vi "Teleop.vi"(10 "Match Info":T1={"Autonomous Elapsed Seconds"=0.0, "TeleOp Elapsed Seconds"=0.0, "Disabled Elapsed Seconds"=0.0, "Visited Autonomous"=FALSE, "Visited TeleOp"=FALSE, "Visited Disabled"=FALSE, "Autonomous Settings"={"Autonomous Style"=enum."Independent", "VI Refnum"=refnum}}, 11 "Call Context":T2) -> ()   [LabVIEW 2016]
doc: "This VI is called for each TeleOp packet received from the DS where the robot is not disabled. It is often used to read from the joysticks and update I/O or to update setpoints for timed control loops. It should complete and return within 20 milliseconds or it may miss DS packets."
uses:
  <vilib>/Rock Robotics/WPI/DriverStation/WPI_DriverStationDerivedRobotMode.ctl
  <vilib>/Rock Robotics/WPI/DriverStation/WPI_DriverStationMatch Info.ctl
  <vilib>/Rock Robotics/WPI/Solenoid/WPI_SolenoidValue.ctl
  <vilib>/Rock Robotics/Network Tables/NT Read Boolean.vi
  <vilib>/Rock Robotics/Network Tables/NT Read Number.vi
  <vilib>/Rock Robotics/WPI/Utilities/WPI_GetSetVariantRefNum.vi
  <vilib>/Rock Robotics/WPI/Solenoid/WPI_SolenoidSetEnum.vi
panel:
  out "Teleop Time Elipsed":dbl
  in  "Quand arreter compresseur":dbl
  out "Droit":dbl
  out "Gauche":dbl
  out "Corde start time":dbl
  out "Sample Slider 0":dbl(slide) scale=0.0..5.0
  out "Sample Boolean 1":bool
  out "Sample Boolean 0":bool
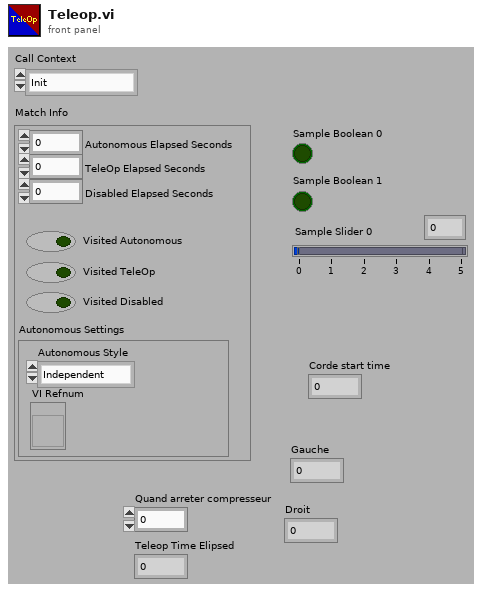
[diagram p1: front panel]
types:
  T1 = typedef "WPI_DriverStationMatch Info.ctl" = cluster{"Autonomous Elapsed Seconds":dbl, "TeleOp Elapsed Seconds":dbl, "Disabled Elapsed Seconds":dbl, "Visited Autonomous":bool, "Visited TeleOp":bool, "Visited Disabled":bool, "Autonomous Settings":cluster{"Autonomous Style":enum16{"Iterative", "Independent"}, "VI Refnum":refnum<vi>}}
  T2 = typedef "WPI_DriverStationDerivedRobotMode.ctl" = enum16{"Init", "Execute", "Stop"}
  T3 = typedef "WPI_SolenoidValue.ctl" = enum16{"Off", "On", "Forward", "Reverse"}
  T4 = typedef "WPI_JoystickDevRef.ctl" = cluster{"Device":T5}
  T5 = typedef "WPI_JoystickDeviceEnum.ctl" = enum16{"USB 0", "USB 1", "USB 2", "USB 3", "USB 4", "USB 5"}
  T6 = typedef "WPI_EncoderDevRef.ctl" = cluster{"DevStatus":errorcluster, "EncoderIndex":T7, "CounterIndex":T8, "DistancePerCount":dbl, "Decoding Type":T9}
  T7 = typedef "FPGA_EncoderIdx.ctl" = enum8{"Enc 0", "Enc 1", "Enc 2", "Enc 3", "Enc 4", "Enc 5", "Enc 6", "Enc 7", "Invalid"}
  T8 = typedef "FPGA_CounterCtrSystemIndex.ctl" = enum8{"Ctr 0", "Ctr 1", "Ctr 2", "Ctr 3", "Ctr 4", "Ctr 5", "Ctr 6", "Ctr 7", "Invalid"}
  T9 = typedef "WPI_EncoderType.ctl" = enum16{"1x", "2x", "4x"}
  T10 = cluster{"Buttons[0]":bool, "Buttons[1]":bool, "Buttons[2]":bool, "Buttons[3]":bool, "Buttons[4]":bool, "Buttons[5]":bool, "Buttons[6]":bool, "Buttons[7]":bool, "Buttons[8]":bool}
  T11 = cluster{"Axes[0]":dbl, "Axes[1]":dbl, "Axes[2]":dbl, "Axes[3]":dbl, "Axes[4]":dbl, "Axes[5]":dbl, "Axes[6]":dbl, "Axes[7]":dbl, "Axes[8]":dbl}
  T12 = typedef "WPI_RobotDriveDevRef.ctl" = cluster{"DevStatus":errorcluster, "Motors[]":T13[], "Square Inputs":bool, "Max Output":dbl}
  T13 = typedef "WPI_MotorControlDeviceRef.ctl" = cluster{"DeviceStatus":errorcluster, "Type":T14, "PWM":cluster{"PWM Channel":T15, "DeadBand":T16}, "CAN":cluster{"Device Number":u8, "SetOutput VI Ref":variant, "GetOutput VI Ref":variant, "Enable VI Ref":variant, "Disable VI Ref":variant, "Data":variant}, "Invert":bool}
  T14 = typedef "WPI_MotorControlType.ctl" = enum16{"PWM", "CAN"}
  T15 = typedef "FPGA_DIOPWMChannel.ctl" = enum8{"PWM 0", "PWM 1", "PWM 2", "PWM 3", "PWM 4", "PWM 5", "PWM 6", "PWM 7", "PWM 8", "PWM 9", "PWM MXP 0", "PWM MXP 1", "PWM MXP 2", "PWM MXP 3", "PWM MXP 4", "PWM MXP 5", "PWM MXP 6", "PWM MXP 7", "PWM MXP 8", "PWM MXP 9", "Invalid"}
  T16 = typedef "WPI_PWMDeadband.ctl" = cluster{"Name":string, "maxPositivePwm":i32, "minPositivePwm":i32, "centerPwm":i32, "maxNegativePwm":i32, "minNegativePwm":i32, "angularRange":u16}
  T17 = typedef "WPI_SolenoidDevRef.ctl" = cluster{"DevStatus":errorcluster, "Pneumatics Control Module":u8, "Forward Solenoid Channel":T18, "Reverse Solenoid Channel":T18}
  T18 = typedef "WPI_SolenoidChannel.ctl" = enum8{"Solenoid 0", "Solenoid 1", "Solenoid 2", "Solenoid 3", "Solenoid 4", "Solenoid 5", "Solenoid 6", "Solenoid 7", "Invalid"}
  T19 = typedef "WPI_CompressorDevRef.ctl" = cluster{"DevStatus":errorcluster, "Pneumatics Control Module":u8}
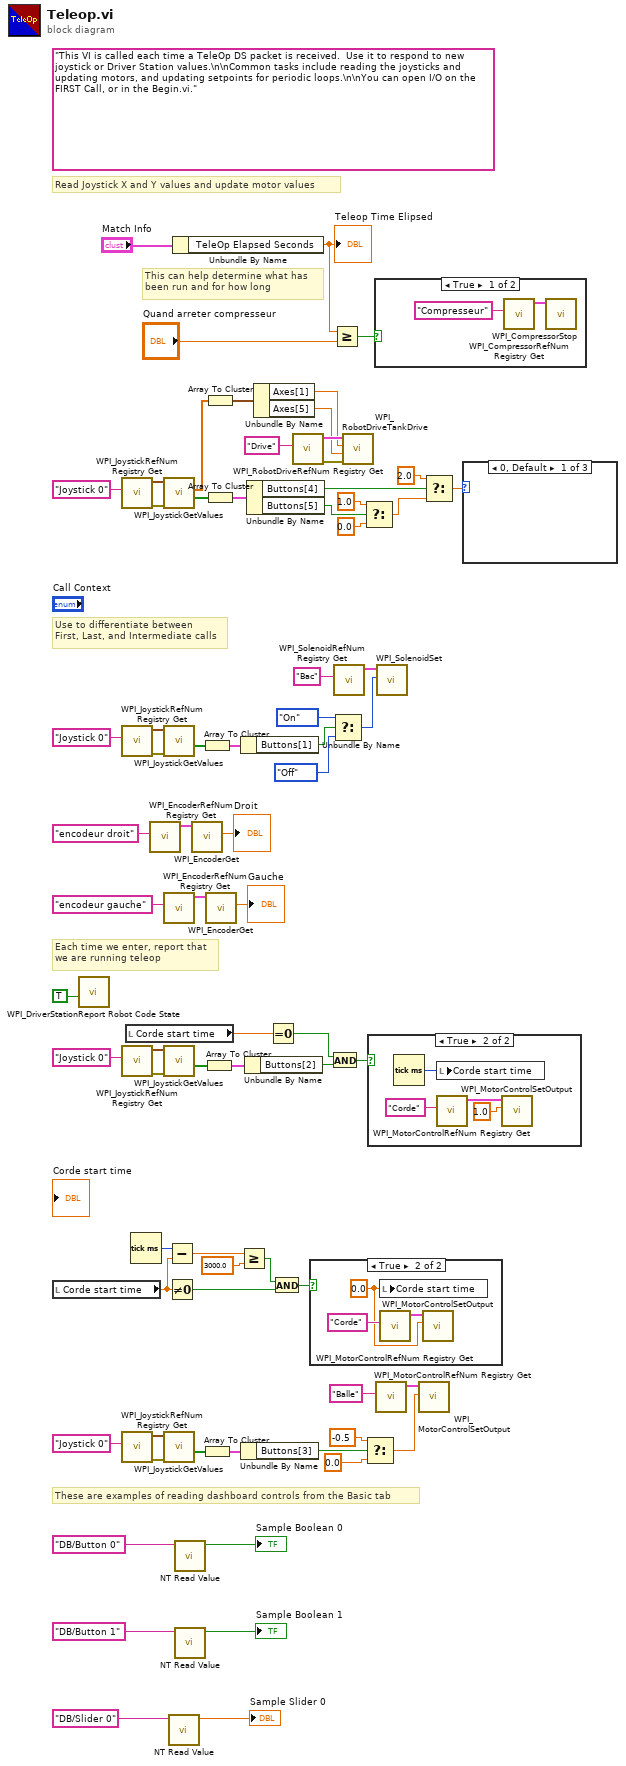
[diagram p0: block diagram]
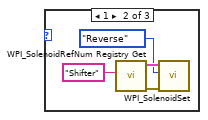
[diagram p5: hidden frame]
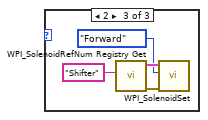
[diagram p6: hidden frame]
diagram:
  (unwired) "This VI is called each time a TeleOp DS packet is received.  Use it to respond to new joystick or Driver Station values.\n\nCommon tasks include reading the joysticks and updating motors, and updating setpoints for periodic loops.\n\nYou can open I/O on the FIRST Call, or in the Begin.vi."
  # "These are examples of reading dashboard controls from the Basic tab"
  # "Each time we enter, report that\nwe are running teleop"
  # "Use to differentiate between\nFirst, Last, and Intermediate calls"
  # "This can help determine what has\nbeen run and for how long"
  # "Read Joystick X and Y values and update motor values"
  n1 = local read "Corde start time"() -> (w10:dbl)
  n2 = call <vilib>:"WPI_DriverStationReport Robot Code State.vi"("TeleOp"=TRUE ("Autonomous")) -> ()  [unwired: 10 in, 1 out]
  n3 = call <vilib>:"WPI_JoystickRefNum Registry Get.vi"("refnum name"="Joystick 0") -> ("error out"=w63:errorcluster, "JoystickDevRef"=w62:T4)  [unwired: 9 in]
  n4 = call <vilib>:"WPI_JoystickRefNum Registry Get.vi"("refnum name"="Joystick 0") -> ("error out"=w47:errorcluster, "JoystickDevRef"=w48:T4)  [unwired: 1 in, 8 out]
  n5 = call <vilib>:"WPI_JoystickRefNum Registry Get.vi"("refnum name"="Joystick 0") -> ("error out"=w36:errorcluster, "JoystickDevRef"=w37:T4)  [unwired: 1 in, 8 out]
  n6 = call <vilib>:"WPI_JoystickRefNum Registry Get.vi"("refnum name"="Joystick 0") -> ("error out"=w31:errorcluster, "JoystickDevRef"=w32:T4)  [unwired: 1 in, 8 out]
  n7 = local read "Corde start time"() -> (w17:dbl)
  n8 = Tick Count (ms)() -> (millisecond timer value=w16:u32)
  n9 = call <vilib>:"WPI_EncoderRefNum Registry Get.vi"("refnum name"="encodeur droit") -> ("EncoderDevRef"=w8:T6)  [unwired: 9 in, 1 out]
  n10 = call <vilib>:"WPI_JoystickGetValues.vi"("error in (no error)"=w63, "JoystickDevRef"=w62) -> ("Buttons"=w58:bool[], "Axes"=w61:dbl[])  [unwired: 5 in, 3 out]
  n11 = call <vilib>:"WPI_JoystickGetValues.vi"("error in (no error)"=w47, "JoystickDevRef"=w48) -> ("Buttons"=w46:bool[])  [unwired: 5 in, 4 out]
  n12 = call <vilib>:"WPI_EncoderRefNum Registry Get.vi"("refnum name"="encodeur gauche") -> ("EncoderDevRef"=w9:T6)  [unwired: 9 in, 1 out]
  n13 = call <vilib>:"WPI_JoystickGetValues.vi"("error in (no error)"=w36, "JoystickDevRef"=w37) -> ("Buttons"=w35:bool[])  [unwired: 5 in, 4 out]
  n14 = call <vilib>:"WPI_JoystickGetValues.vi"("error in (no error)"=w31, "JoystickDevRef"=w32) -> ("Buttons"=w30:bool[])  [unwired: 5 in, 4 out]
  n15 = Subtract(x=w16, y=w10) -> (x-y=w15:dbl)
  n16 = Not Equal To 0?(x=w10) -> (x != 0?=w12:bool)
  n17 = call-poly <vilib>:"NT Read Value.vi"("Name"="DB/Slider 0" ("refnum name")) -> ("Numeric"=→"Sample Slider 0":dbl)  [unwired: 9 in, 1 out]
  n18 = Unbundle By Name("Match Info") -> ("TeleOp Elapsed Seconds"=w1:dbl)
  "Teleop Time Elipsed" <- w1
  n19 = call-poly <vilib>:"NT Read Value.vi"("Name"="DB/Button 0" ("refnum name")) -> ("Boolean"=→"Sample Boolean 0":bool)  [unwired: 9 in, 1 out]
  n20 = call-poly <vilib>:"NT Read Value.vi"("Name"="DB/Button 1" ("refnum name")) -> ("Boolean"=→"Sample Boolean 1":bool)  [unwired: 9 in, 1 out]
  n21 = call <vilib>:"WPI_EncoderGet.vi"("EncoderDevRef"=w8) -> ("Distance"=→"Droit":dbl)  [unwired: 5 in, 5 out]
  n22 = Array To Cluster(array=w46) -> (cluster=w45:T10)
  n23 = Array To Cluster(array=w30) -> (cluster=w29:T10)
  n24 = Array To Cluster(array=w35) -> (cluster=w34:T10)
  n25 = Array To Cluster(array=w61) -> (cluster=w60:T11)
  n26 = Array To Cluster(array=w58) -> (cluster=w57:T10)
  n27 = call <vilib>:"WPI_EncoderGet.vi"("EncoderDevRef"=w9) -> ("Distance"=→"Gauche":dbl)  [unwired: 5 in, 5 out]
  n28 = Greater Or Equal?(x=w15, y=3000.0) -> (x >= y?=w11:bool)
  n29 = Unbundle By Name(w45) -> ("Buttons[1]"=w44:bool)
  n30 = Unbundle By Name(w29) -> ("Buttons[3]"=w28:bool)
  n31 = Unbundle By Name(w34) -> ("Buttons[2]"=w19:bool)
  n32 = Unbundle By Name(w57) -> ("Buttons[4]"=w56:bool, "Buttons[5]"=w52:bool)
  n33 = Unbundle By Name(w60) -> ("Axes[1]"=w22:dbl, "Axes[5]"=w21:dbl)
  n34 = Equal To 0?(x=w17) -> (x = 0?=w18:bool)
  n35 = And(x=w11, y=w12) -> (x .and. y?=w13:bool)
  n36 = call <vilib>:"WPI_RobotDriveRefNum Registry Get.vi"("refnum name"="Drive") -> ("error out"=w66:errorcluster, "RobotDriveDevRef"=w65:T12)  [unwired: 9 in]
  n37 = case shown="True" w13 {
    frame False {
    }
    frame True {
      w75 = 0.0 ("Corde start time")
      n38 = local write "Corde start time"(w75) -> ()
      n39 = call <vilib>:"WPI_MotorControlRefNum Registry Get.vi"("refnum name"="Corde") -> ("MotorControlDevRef"=w77:T13)  [unwired: 9 in, 1 out]
      n40 = call <vilib>:"WPI_MotorControlSetOutput.vi"("Output"=w75, "MotorControlDevRef"=w77) -> ()  [unwired: 7 in, 3 out]
    }
  }
  n41 = And(x=w18, y=w19) -> (x .and. y?=w20:bool)
  n42 = Greater Or Equal?(x=w1, y="Quand arreter compresseur") -> (x >= y?=w2:bool)
  n43 = Select(t=WPI_SolenoidValue."On" ("Value"), s=w44, f=WPI_SolenoidValue."Off" ("Value")) -> (s? t:f=w39:T3)
  n44 = call <vilib>:"WPI_SolenoidRefNum Registry Get.vi"("refnum name"="Bac") -> ("SolenoidDevRef"=w40:T17)  [unwired: 9 in, 1 out]
  n45 = call <vilib>:"WPI_RobotDriveTankDrive.vi"("error in (no error)"=w66, "Right axis value"=w21, "Left axis value"=w22, "RobotDriveDevRef"=w65) -> ()  [unwired: 5 in, 3 out]
  n46 = Select(t=1.0, s=w52, f=0.0) -> (s? t:f=w54:dbl)
  n47 = Select(t=-0.5, s=w28, f=0.0) -> (s? t:f=w25:dbl)
  n48 = case shown="True" w20 {
    frame False {
    }
    frame True {
      n49 = Tick Count (ms)() -> (millisecond timer value=w81:u32)
      n50 = local write "Corde start time"(w81) -> ()
      n51 = call <vilib>:"WPI_MotorControlRefNum Registry Get.vi"("refnum name"="Corde") -> ("MotorControlDevRef"=w80:T13)  [unwired: 9 in, 1 out]
      n52 = call <vilib>:"WPI_MotorControlSetOutput.vi"("Output"=1.0, "MotorControlDevRef"=w80) -> ()  [unwired: 7 in, 3 out]
    }
  }
  n53 = case shown="True" w2 {
    frame True {
      n54 = call <vilib>:"WPI_CompressorRefNum Registry Get.vi"("refnum name"="Compresseur") -> ("CompressorDevRef"=w83:T19)  [unwired: 9 in, 1 out]
      n55 = call <vilib>:"WPI_CompressorStop.vi"("CompressorDevRef"=w83) -> ()  [unwired: 9 in, 2 out]
    }
    frame False {
    }
  }
  n56 = call <vilib>:"WPI_MotorControlRefNum Registry Get.vi"("refnum name"="Balle") -> ("MotorControlDevRef"=w23:T13)  [unwired: 9 in, 1 out]
  n57 = call-poly <vilib>:"WPI_SolenoidSet.vi"("Value"=w39, "SolenoidDevRef"=w40) -> ()  [unwired: 8 in, 2 out]
  n58 = call <vilib>:"WPI_MotorControlSetOutput.vi"("Output"=w25, "MotorControlDevRef"=w23) -> ()  [unwired: 7 in, 3 out]
  n59 = Select(t=2.0, s=w56, f=w54) -> (s? t:f=w50:dbl)
  n60 = case shown="0, Default" w50 {
    frame 0, Default {
    }
    frame 1 {
      n61 = call <vilib>:"WPI_SolenoidRefNum Registry Get.vi"("refnum name"="Shifter") -> ("error out"=w86:errorcluster, "SolenoidDevRef"=w85:T17)  [unwired: 9 in]
      n62 = call-poly <vilib>:"WPI_SolenoidSet.vi"("error in (no error)"=w86, "Value"=WPI_SolenoidValue."Reverse", "SolenoidDevRef"=w85) -> ()  [unwired: 7 in, 2 out]
    }
    frame 2 {
      n63 = call <vilib>:"WPI_SolenoidRefNum Registry Get.vi"("refnum name"="Shifter") -> ("error out"=w90:errorcluster, "SolenoidDevRef"=w89:T17)  [unwired: 9 in]
      n64 = call-poly <vilib>:"WPI_SolenoidSet.vi"("error in (no error)"=w90, "Value"=WPI_SolenoidValue."Forward", "SolenoidDevRef"=w89) -> ()  [unwired: 7 in, 2 out]
    }
  }
